vi "test - LabVIEW-Config.vi"(8 "error in (no error)":errorcluster, 11 "TestCase in":refnum<class "labview-config-library.lvclass">) -> (0 "error out":errorcluster, 3 "TestCase out":refnum<class "labview-config-library.lvclass">)   [LabVIEW 2017, in "labview-config-library.lvclass"]
uses:
  labview-config-library.lvclass
  <vilib>/addons/_JKI Toolkits/VI Tester/TestCase.llb/TestCase.lvclass
  C:/Program Files (x86)/National Instruments/LabVIEW 2017/vi.lib/addons/_JKI Toolkits/VI Tester/TestCase.llb/TestCase.lvclass
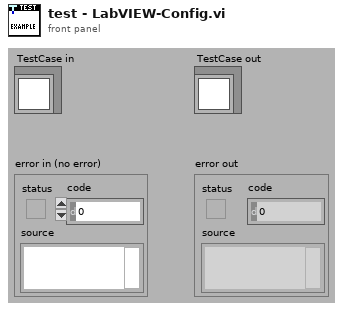
[diagram p1: front panel]
types:
  T1 = cluster{"String":string, "Boolean":bool, "Int":i32, "Uint":u32, "Float":dbl, "Raw":string}
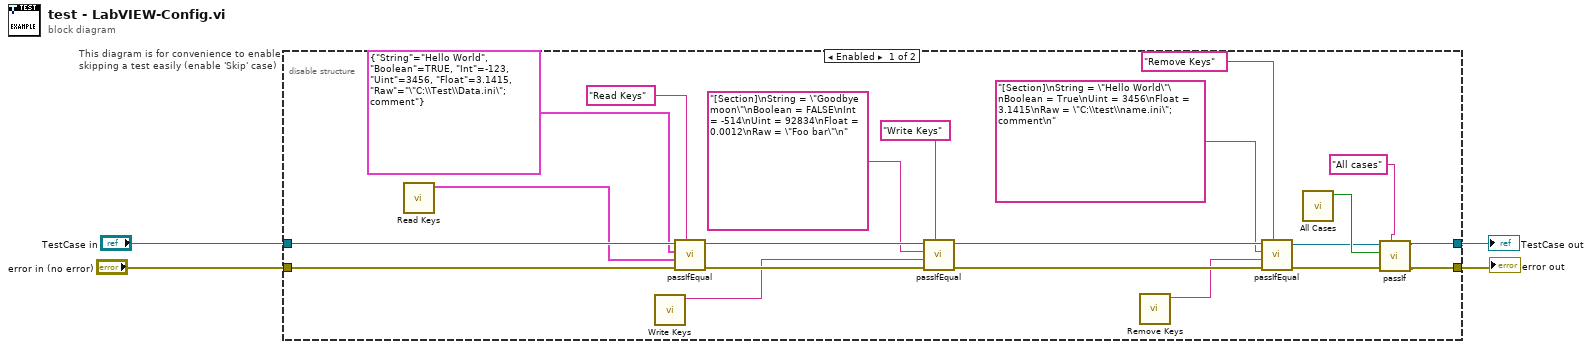
[diagram p0: block diagram]
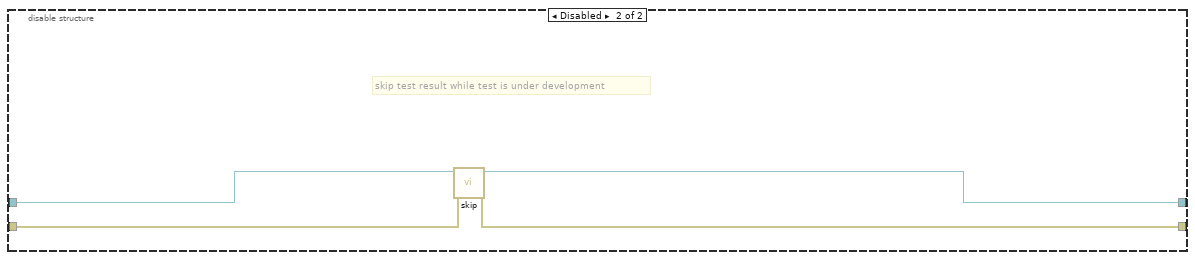
[diagram p2: hidden frame]
diagram:
  n1 = disable-structure "This diagram is for convenience to enable skipping a test easily (enable 'Skip' case)" shown="Enabled" {
    disable-tunnel: "TestCase in" -> [w21 w29]
    disable-tunnel: [w25 w27] -> w1
    disable-tunnel: [w24 w28] -> w3
    disable-tunnel: "error in (no error)" -> [w20 w26]
    frame Enabled {
      n2 = call "Read Keys.vi"() -> ("Config"=w18:T1)  [unwired: 10 in, 1 out]
      n3 = call "Write Keys.vi"() -> ("text"=w14:string)  [unwired: 10 in, 1 out]
      n4 = call-dynamic "passIfEqual.vi"("custom report message (\"\")"="Read Keys" ("custom report message (\"\")"), "error in (no error)"=w20, "y"=w18, "x"=T1 {"String"="Hello World", "Boolean"=TRUE, "Int"=-123, "Uint"=3456, "Float"=3.1415, "Raw"="\"C:\\Test\\Data.ini\"; comment"} ("Config"), "TestCase in"=w21) -> ("error out"=w16:errorcluster, "TestCase out"=w15:refnum<class "labview-config-library.lvclass">)  [unwired: 5 in]
      n5 = call-dynamic "passIfEqual.vi"("custom report message (\"\")"="Write Keys" ("custom report message (\"\")"), "error in (no error)"=w16, "y"=w14, "x"="[Section]\nString = \"Goodbye moon\"\nBoolean = FALSE\nInt = -514\nUint = 92834\nFloat = 0.0012\nRaw = \"Foo bar\"\n" ("text"), "TestCase in"=w15) -> ("error out"=w8:errorcluster, "TestCase out"=w9:refnum<class "labview-config-library.lvclass">)  [unwired: 5 in]
      n6 = call "Remove Keys.vi"() -> ("text"=w6:string)  [unwired: 10 in, 1 out]
      n7 = call-dynamic "passIfEqual.vi"("custom report message (\"\")"="Remove Keys" ("custom report message (\"\")"), "error in (no error)"=w8, "y"=w6, "x"="[Section]\nString = \"Hello World\"\nBoolean = True\nUint = 3456\nFloat = 3.1415\nRaw = \"C:\\test\\name.ini\"; comment\n" ("text"), "TestCase in"=w9) -> ("error out"=w10:errorcluster, "TestCase out"=w11:refnum<class "labview-config-library.lvclass">)  [unwired: 5 in]
      n8 = call "All Cases.vi"() -> ("All Passed"=w23:bool)  [unwired: 10 in, 1 out]
      n9 = call-dynamic "passIf.vi"("custom report message (\"\")"="All cases" ("custom report message (\"\")"), "error in (no error)"=w10, "pass"=w23, "TestCase in"=w11) -> ("error out"=w24:errorcluster, "TestCase out"=w25:refnum<class "labview-config-library.lvclass">)  [unwired: 6 in]
    }
    frame Disabled {
      # "skip test result while test is under development"
      n10 = call <vilib>:"skip.vi"("error in (no error)"=w26, "TestCase in"=w29) -> ("error out"=w28:errorcluster, "TestCase out"=w27:refnum<class "labview-config-library.lvclass">)  [unwired: 8 in]
    }
  }
  "error out" <- w3
  "TestCase out" <- w1
